vi "Set Slit Width.vi"(8 "error in (no error)":errorcluster, 9 "Slit":T1, 10 "Slit Width (um)":dbl, 11 "Simulated in":refnum<class "Simulated.lvclass">) -> (0 "error out":errorcluster, 2 "Slit Width (um) out":dbl, 3 "Simulated out":refnum<class "Simulated.lvclass">)   [LabVIEW 2019, in "Simulated.lvclass"]
uses:
  Simulated.lvclass
  Types/Slit.ctl
  Simulated.lvclass/Simulated.ctl
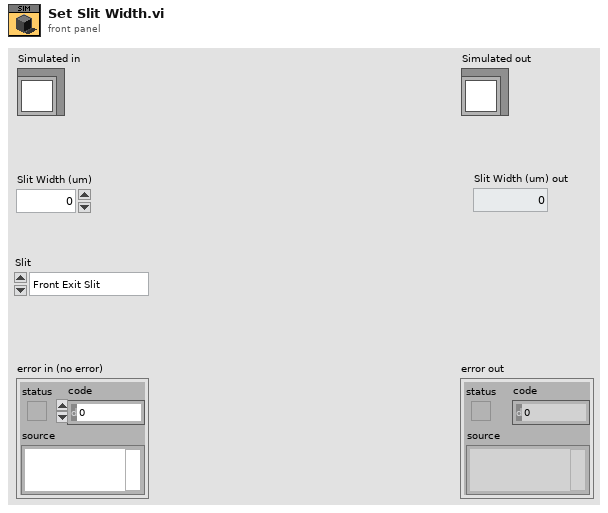
[diagram p1: front panel]
types:
  T1 = typedef "Slit.ctl" = enum16{"Front Exit Slit", "Side Exit Slit", "Front Entrance Slit", "Side Entrance Slit"}
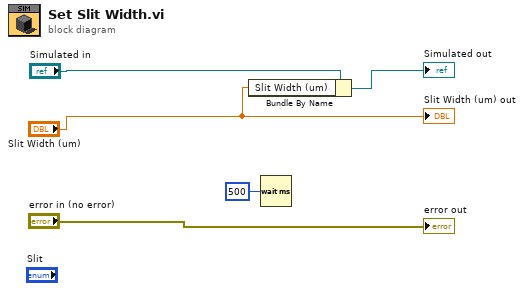
[diagram p0: block diagram]
diagram:
  n1 = Bundle By Name(cluster="Simulated in", "Slit Width (um)"="Slit Width (um)") -> (→"Simulated out":refnum<class "Simulated.lvclass">)
  n2 = Wait (ms)(milliseconds to wait=u32 500) -> ()  [unwired: 1 out]
  "error out" <- "error in (no error)"
  "Slit Width (um) out" <- "Slit Width (um)"
